vi "Rename VIs.vi"(8 "error in (no error)":errorcluster, 11 "ProjectItem in":refnum<class "ProjectItem.lvclass">) -> (0 "error out":errorcluster, 3 "ProjectItem out":refnum<class "ProjectItem.lvclass">)   [LabVIEW 2019, in "ProjectItem.lvclass"]
uses:
  ProjectItem.lvclass
  ProjectItem.lvclass/ProjectItem.ctl
panel:
  out "VI Names":string[](array[string])
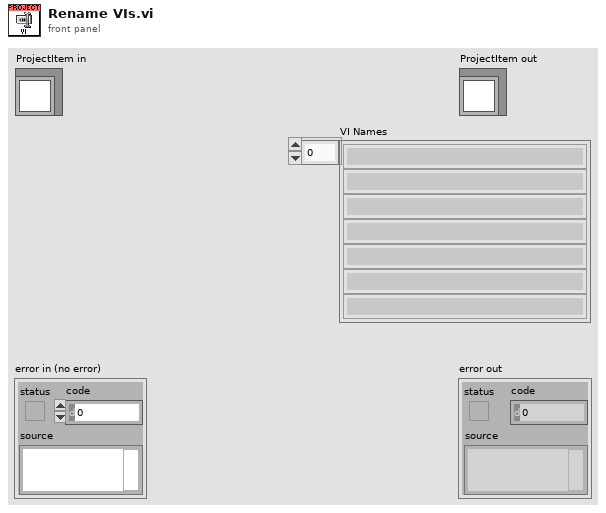
[diagram p1: front panel]
types:
  T1 = cluster{"Class":refnum<vi>, "DynamicVIs":refnum<vi>[], "StaticVIs":refnum<vi>[], "Name":string, "Icon":refnum<class "Icon.lvclass">}[]
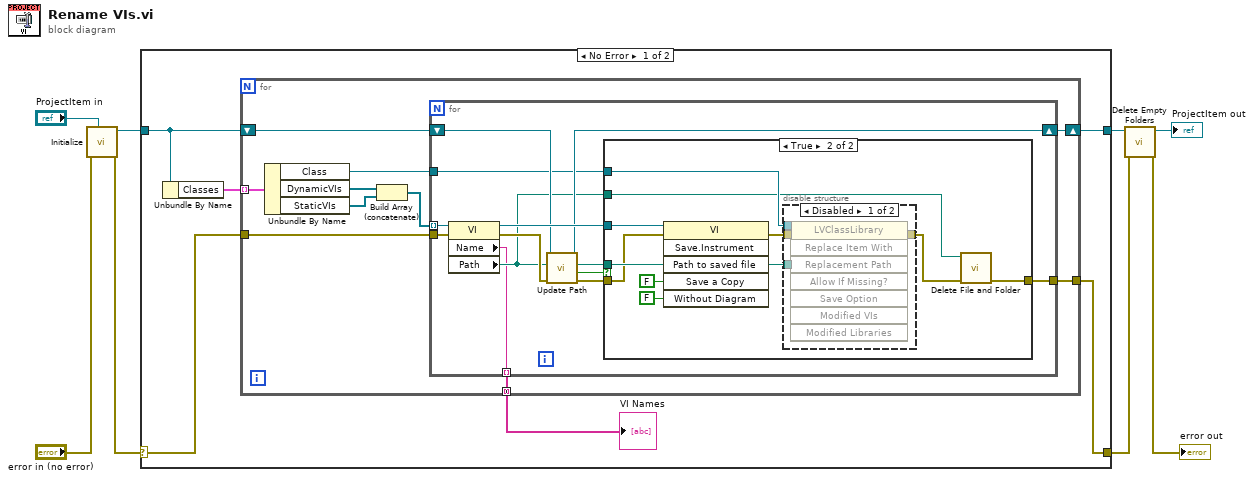
[diagram p0: block diagram]
diagram:
  n1 = call "Initialize.vi"("ProjectItem"="ProjectItem in", "error in (no error)"="error in (no error)") -> ("error out"=w5:errorcluster, "ProjectItem out"=w7:refnum<class "ProjectItem.lvclass">)  [unwired: 8 in]
  n2 = case shown="No Error" w5 {
    selector: w5 -> [w13 w55]
    tunnel: [w10 w55] -> w2
    tunnel: [w14 w54] -> w4
    tunnel: w7 -> [w11 w54]
    frame No Error {
      n3 = Unbundle By Name(w11) -> ("Classes"=w12:T1)
      n4 = for {
        tunnel: w13 -> [w24]
        shift-right: [w23] -> w14
        shift-left: w11 -> [w22]
        tunnel: w12 -> [w21] mode=indexing
        tunnel: [w16] -> w10
        tunnel: [w15] -> w9 mode=concatenating
        n5 = Unbundle By Name(w21) -> ("Class"=w18:refnum<vi>, "DynamicVIs"=w20:refnum<vi>[], "StaticVIs"=w19:refnum<vi>[])
        n6 = Build Array (concatenate)(w20, w19) -> (w17:refnum<vi>[])
        n7 = for {
          tunnel: w24 -> [w34]
          shift-right: [w31] -> w23
          shift-left: w22 -> [w33]
          tunnel: w17 -> [w30] mode=indexing
          tunnel: w18 -> [w29]
          tunnel: [w26] -> w16
          tunnel: [w25] -> w15 mode=indexing
          n8 = property class="VI"(reference=w30, error in=w34) -> (reference out=w37:refnum<vi>, error out=w36:errorcluster, "Name"=w25:string, "Path"=w27:path)
          n9 = call "Update Path.vi"("error in (no error)"=w36, "Path in"=w27, "Rename in"=w33) -> ("error out"=w35:errorcluster, "New Path?"=w28:bool, "Path out"=w32:path, "Rename out"=w31:refnum<class "ProjectItem.lvclass">)  [unwired: 5 in]
          n10 = case shown="True" w28 {
            tunnel: w37 -> [_ w48]
            tunnel: w35 -> [w38 w43]
            tunnel: w32 -> [_ w45]
            tunnel: w29 -> [_ w44]
            tunnel: w27 -> [_ w39]
            tunnel: [w38 w40] -> w26
            frame False {
            }
            frame True {
              n11 = invoke class="VI" method="Save.Instrument"(reference=w48, error in=w43, "Path to saved file"=w45, "Save a Copy"=FALSE, "Without Diagram"=FALSE) -> (error out=w41:errorcluster)  [unwired: 1 in, 5 out]
              n12 = disable-structure shown="Disabled" {
                disable-tunnel: w45 -> [w52 _]
                disable-tunnel: w44 -> [w51 _]
                disable-tunnel: [w50 w53] -> w42
                disable-tunnel: w41 -> [w49 w53]
                frame Disabled {
                  n13 = invoke class="LVClassLibrary" method="Replace Item With"(reference=w51, error in=w49, "Replacement Path"=w52) -> (error out=w50:errorcluster)  [unwired: 5 in, 7 out]
                }
                frame Enabled {
                }
              }
              n14 = call "Delete File and Folder.vi"("error in (no error)"=w42, "Path"=w39) -> ("error out"=w40:errorcluster)  [unwired: 9 in]
            }
          }
        }
      }
      "VI Names" <- w9
    }
    frame Error {
    }
  }
  n15 = call "Delete Empty Folders.vi"("error in (no error)"=w2, "Rename in"=w4) -> ("error out"=→"error out":errorcluster, "Rename out"=→"ProjectItem out":refnum<class "ProjectItem.lvclass">)  [unwired: 8 in]
